vi "Register for Event.vi"(4 "Error In":errorcluster) -> (0 "Error Out":errorcluster, 3 "daq":refnum<event-registration>)   [LabVIEW 2014, in "Change Source.lvlib"]
uses:
  Change Source.lvlib
  _typedefs/Event Data.ctl
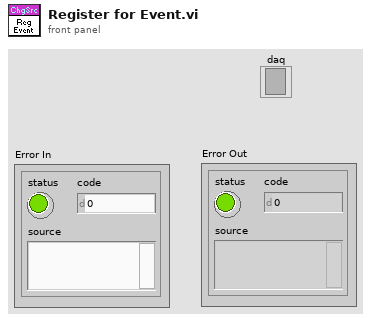
[diagram p1: front panel]
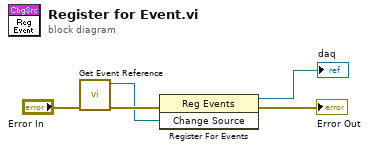
[diagram p0: block diagram]
diagram:
  n1 = call "Get Event Reference.vi"("error in (no error)"="Error In") -> ("error out"=w4:errorcluster, "Change Source"=w3:refnum<user-event>)  [unwired: 5 in]
  n2 = register-events(error in=w4, w3) -> (reference out=→"daq":refnum<event-registration>, error out=→"Error Out":errorcluster)  [unwired: 1 in]
